vi "Autonomous Mode.vi"(0 "Drive Motors":string="RobotDrive", 1 "Ball Holders":string="RobotDrive", 5 "B.Pick up":string="My Motor RefNum", 7 "A.Pick up":string="My Solenoid RefNum", 9 "Shooter":string="My Motor RefNum", 11 "Inverted Shooter":string="My Motor RefNum") -> ()   [LabVIEW 2013]
uses:
  <vilib>/Rock Robotics/WPI/Solenoid/WPI_SolenoidValue.ctl
  <vilib>/Rock Robotics/WPI/RobotDrive/WPI_RobotDriveGetSetRefNum.vi
  <vilib>/Rock Robotics/WPI/Solenoid/Deprecated/WPI_SolenoidGetBool.vi
  <vilib>/Rock Robotics/WPI/Solenoid/WPI_SolenoidSetEnum.vi
  Ultrasonic Sensor.vi
  <vilib>/Rock Robotics/WPI/RobotDrive/WPI_RobotDriveArcadeDrive_Standard(NoSaturation).vi
panel:
  in  "Auton Shot 2":string="AUTON-Shot"
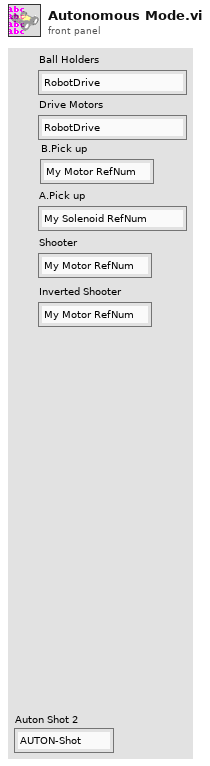
[diagram p1: front panel]
types:
  T1 = typedef "WPI_MotorControlDeviceRef.ctl" = cluster{"DeviceStatus":errorcluster, "Type":enum16{"PWM", "CAN"}, "PWM":cluster{"Digital Module":T2, "PWM Channel":T3, "DeadBand":T4}, "CAN":cluster{"Device Number":u8, "Control Mode":T5, "Semaphore":T6, "Max Vout":dbl}, "Invert":bool, "TransformRef":T7, "InvTransformRef":T7}
  T2 = typedef "FPGA_TypedefDigitalModule.ctl" = enum16{"Digital Module 1", "Digital Module 2"}
  T3 = typedef "FPGA_DIOPWMChannel.ctl" = enum8{"PWM 1", "PWM 2", "PWM 3", "PWM 4", "PWM 5", "PWM 6", "PWM 7", "PWM 8", "PWM 9", "PWM 10", "Invalid"}
  T4 = typedef "WPI_PWMDeadband.ctl" = cluster{"Name":string, "maxPositivePwm":i32, "minPositivePwm":i32, "centerPwm":i32, "maxNegativePwm":i32, "minNegativePwm":i32, "angularRange":u16}
  T5 = typedef "WPI_CANJaguar_ControlMode.ctl" = enum8{"Percent VBus", "Current", "Speed", "Position", "Voltage"}
  T6 = typedef "Semaphore RefNum" = refnum<k1>
  T7 = typedef "WPI_PWMTransform_ConPane.ctl" = refnum<vi>
  T8 = typedef "WPI_SolenoidDevRef.ctl" = cluster{"DevStatus":errorcluster, "Solenoid Module":T9, "Forward Solenoid Channel":T10, "Reverse Solenoid Channel":T10}
  T9 = typedef "FPGA_TypedefSolenoidModule.ctl" = enum16{"Solenoid Module 1", "Solenoid Module 2"}
  T10 = typedef "WPI_SolenoidChannel.ctl" = enum8{"Solenoid 1", "Solenoid 2", "Solenoid 3", "Solenoid 4", "Solenoid 5", "Solenoid 6", "Solenoid 7", "Solenoid 8", "Invalid"}
  T11 = typedef "WPI_RobotDriveDevRef.ctl" = cluster{"DevStatus":errorcluster, "Motors[]":T1[], "Square Inputs":bool, "Max Output":dbl, "Isochronous":bool}
  T12 = typedef "WPI_SolenoidValue.ctl" = enum16{"Off", "On", "Forward", "Reverse"}
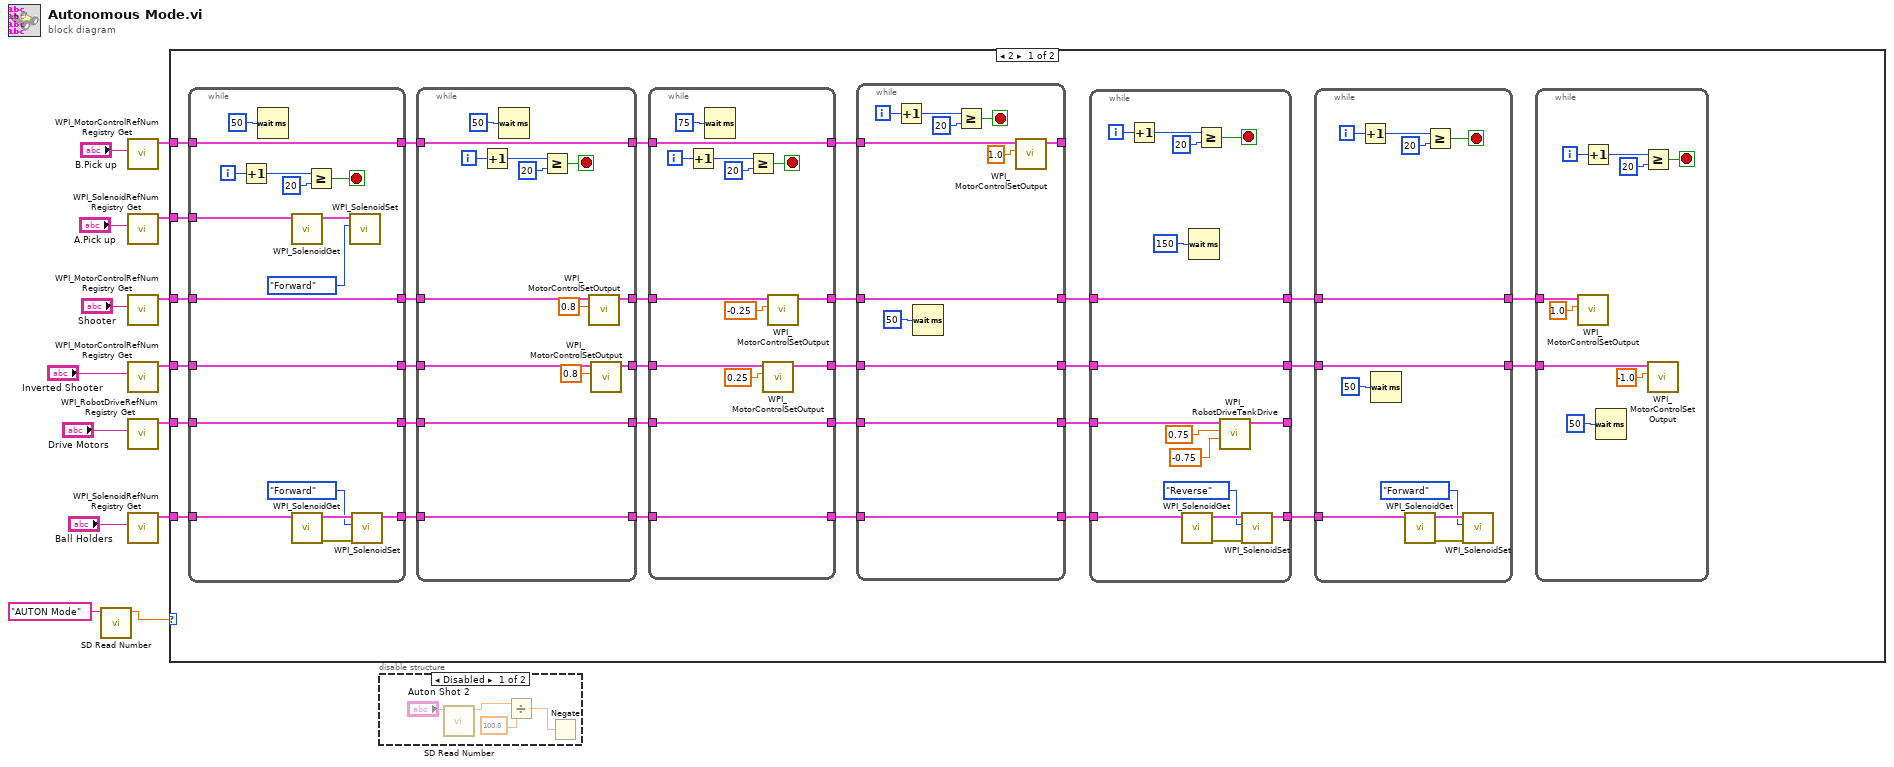
[diagram p0: block diagram]
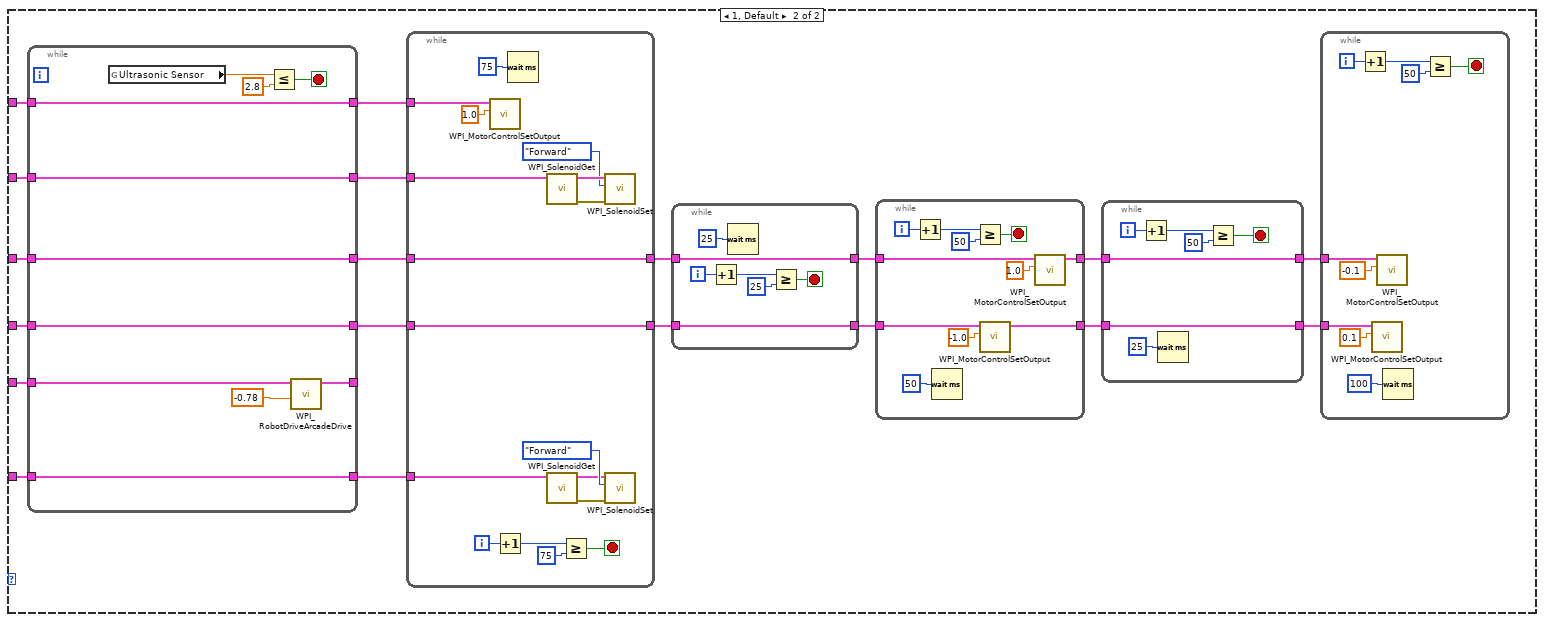
[diagram p3: hidden frame]
diagram:
  n1 = call <vilib>:"SD Read Number.vi"("Name"="AUTON Mode") -> ("Numeric"=w2:dbl)  [unwired: 8 in, 2 out]
  n2 = call <vilib>:"WPI_MotorControlRefNum Registry Get.vi"("refnum name"="B.Pick up") -> ("MotorControlDevRef"=w5:T1)  [unwired: 9 in, 1 out]
  n3 = call <vilib>:"WPI_SolenoidRefNum Registry Get.vi"("refnum name"="A.Pick up") -> ("SolenoidDevRef"=w11:T8)  [unwired: 9 in, 1 out]
  n4 = call <vilib>:"WPI_MotorControlRefNum Registry Get.vi"("refnum name"="Shooter") -> ("MotorControlDevRef"=w7:T1)  [unwired: 9 in, 1 out]
  n5 = call <vilib>:"WPI_MotorControlRefNum Registry Get.vi"("refnum name"="Inverted Shooter") -> ("MotorControlDevRef"=w6:T1)  [unwired: 9 in, 1 out]
  n6 = call <vilib>:"WPI_RobotDriveRefNum Registry Get.vi"("refnum name"="Drive Motors") -> ("RobotDriveDevRef"=w14:T11)  [unwired: 9 in, 1 out]
  n7 = call <vilib>:"WPI_SolenoidRefNum Registry Get.vi"("refnum name"="Ball Holders") -> ("SolenoidDevRef"=w3:T8)  [unwired: 9 in, 1 out]
  n8 = case shown="2" w2 {
    tunnel: w14 -> [w42 w156]
    tunnel: w11 -> [w44 w155]
    tunnel: w7 -> [w41 w154]
    tunnel: w6 -> [w40 w153]
    tunnel: w5 -> [w39 w152]
    tunnel: w3 -> [w43 w139]
    frame 2 {
      n9 = while {
        tunnel: w44 -> [w137]
        tunnel: w43 -> [w128]
        tunnel: [w134] -> w35
        tunnel: w42 -> [w134]
        tunnel: [w133] -> w38
        tunnel: w41 -> [w133]
        tunnel: [w132] -> w37
        tunnel: w40 -> [w132]
        tunnel: [w131] -> w36
        tunnel: w39 -> [w131]
        tunnel: [w126] -> w23
        i -> [w125]
        stop <- w124 stop-if-true
        n10 = Increment(x=w125) -> (x+1=w123:i32)
        n11 = Wait (ms)(milliseconds to wait=u32 50) -> ()  [unwired: 1 out]
        n12 = call-poly <vilib>:"WPI_SolenoidGet.vi"("SolenoidDevRef"=w137) -> ("SolenoidDevRef"=w136:T8)  [unwired: 8 in, 2 out]
        n13 = call-poly <vilib>:"WPI_SolenoidGet.vi"("SolenoidDevRef"=w128) -> ("error out"=w130:errorcluster, "SolenoidDevRef"=w129:T8)  [unwired: 8 in, 1 out]
        n14 = Greater Or Equal?(x=w123, y=20) -> (x >= y?=w124:bool)
        n15 = call-poly <vilib>:"WPI_SolenoidSet.vi"("Value"=WPI_SolenoidValue."Forward", "SolenoidDevRef"=w136) -> ()  [unwired: 8 in, 2 out]
        n16 = call-poly <vilib>:"WPI_SolenoidSet.vi"("error in (no error)"=w130, "Value"=WPI_SolenoidValue."Forward", "SolenoidDevRef"=w129) -> ("SolenoidDevRef"=w126:T8)  [unwired: 7 in, 1 out]
      }
      n17 = while {
        tunnel: w38 -> [w120]
        tunnel: w37 -> [w119]
        tunnel: [w118] -> w32
        tunnel: [w117] -> w33
        tunnel: [w116] -> w31
        tunnel: w36 -> [w116]
        tunnel: [w115] -> w34
        tunnel: w35 -> [w115]
        tunnel: [w114] -> w22
        tunnel: w23 -> [w114]
        i -> [w113]
        stop <- w110 stop-if-true
        n18 = Increment(x=w113) -> (x+1=w112:i32)
        n19 = Wait (ms)(milliseconds to wait=u32 50) -> ()  [unwired: 1 out]
        n20 = Greater Or Equal?(x=w112, y=20) -> (x >= y?=w110:bool)
        n21 = call <vilib>:"WPI_MotorControlSetOutput.vi"("Output"=0.8, "MotorControlDevRef"=w120) -> ("MotorControlDevRef"=w117:T1)  [unwired: 7 in, 2 out]
        n22 = call <vilib>:"WPI_MotorControlSetOutput.vi"("Output"=0.8, "MotorControlDevRef"=w119) -> ("MotorControlDevRef"=w118:T1)  [unwired: 7 in, 2 out]
      }
      n23 = while {
        tunnel: w34 -> [w101]
        tunnel: w33 -> [w103]
        tunnel: w32 -> [w104]
        tunnel: w31 -> [w102]
        tunnel: [w102] -> w28
        tunnel: [w101] -> w27
        tunnel: [w100] -> w29
        tunnel: [w99] -> w30
        tunnel: w22 -> [w98]
        tunnel: [w98] -> w21
        i -> [w97]
        stop <- w94 stop-if-true
        n24 = Increment(x=w97) -> (x+1=w96:i32)
        n25 = Wait (ms)(milliseconds to wait=u32 75) -> ()  [unwired: 1 out]
        n26 = Greater Or Equal?(x=w96, y=20) -> (x >= y?=w94:bool)
        n27 = call <vilib>:"WPI_MotorControlSetOutput.vi"("Output"=0.25, "MotorControlDevRef"=w104) -> ("MotorControlDevRef"=w100:T1)  [unwired: 7 in, 2 out]
        n28 = call <vilib>:"WPI_MotorControlSetOutput.vi"("Output"=-0.25, "MotorControlDevRef"=w103) -> ("MotorControlDevRef"=w99:T1)  [unwired: 7 in, 2 out]
      }
      n29 = while {
        tunnel: w30 -> [w89]
        tunnel: w29 -> [w90]
        tunnel: w28 -> [w92]
        tunnel: w27 -> [w88]
        tunnel: [w90] -> w26
        tunnel: [w89] -> w25
        tunnel: [w88] -> w24
        tunnel: [w87] -> _
        tunnel: w21 -> [w86]
        tunnel: [w86] -> w20
        i -> [w85]
        stop <- w82 stop-if-true
        n30 = Increment(x=w85) -> (x+1=w84:i32)
        n31 = Wait (ms)(milliseconds to wait=u32 50) -> ()  [unwired: 1 out]
        n32 = Greater Or Equal?(x=w84, y=20) -> (x >= y?=w82:bool)
        n33 = call <vilib>:"WPI_MotorControlSetOutput.vi"("Output"=1.0, "MotorControlDevRef"=w92) -> ("MotorControlDevRef"=w87:T1)  [unwired: 7 in, 2 out]
      }
      n34 = while {
        tunnel: [w80] -> w17
        tunnel: w26 -> [w80]
        tunnel: w25 -> [w79]
        tunnel: [w79] -> w18
        tunnel: w24 -> [w78]
        tunnel: [w76] -> _
        tunnel: w20 -> [w75]
        tunnel: [w71] -> w19
        i -> [w70]
        stop <- w66 stop-if-true
        n35 = Increment(x=w70) -> (x+1=w69:i32)
        n36 = call-poly <vilib>:"WPI_SolenoidGet.vi"("SolenoidDevRef"=w75) -> ("error out"=w74:errorcluster, "SolenoidDevRef"=w73:T8)  [unwired: 8 in, 1 out]
        n37 = Wait (ms)(milliseconds to wait=u32 150) -> ()  [unwired: 1 out]
        n38 = Greater Or Equal?(x=w69, y=20) -> (x >= y?=w66:bool)
        n39 = call <vilib>:"WPI_RobotDriveTankDrive.vi"("Right axis value"=-0.75, "Left axis value"=0.75 ("X axis value"), "RobotDriveDevRef"=w78) -> ("RobotDriveDevRef"=w76:T11)  [unwired: 6 in, 2 out]
        n40 = call-poly <vilib>:"WPI_SolenoidSet.vi"("error in (no error)"=w74, "Value"=WPI_SolenoidValue."Reverse", "SolenoidDevRef"=w73) -> ("SolenoidDevRef"=w71:T8)  [unwired: 7 in, 1 out]
      }
      n41 = while {
        tunnel: w19 -> [w64]
        tunnel: w18 -> [w60]
        tunnel: w17 -> [w59]
        tunnel: [w60] -> w16
        tunnel: [w59] -> w15
        i -> [w57]
        stop <- w54 stop-if-true
        n42 = Increment(x=w57) -> (x+1=w58:i32)
        n43 = Wait (ms)(milliseconds to wait=u32 50) -> ()  [unwired: 1 out]
        n44 = call-poly <vilib>:"WPI_SolenoidGet.vi"("SolenoidDevRef"=w64) -> ("error out"=w63:errorcluster, "SolenoidDevRef"=w62:T8)  [unwired: 8 in, 1 out]
        n45 = Greater Or Equal?(x=w58, y=20) -> (x >= y?=w54:bool)
        n46 = call-poly <vilib>:"WPI_SolenoidSet.vi"("error in (no error)"=w63, "Value"=WPI_SolenoidValue."Forward", "SolenoidDevRef"=w62) -> ()  [unwired: 7 in, 2 out]
      }
      n47 = while {
        tunnel: w16 -> [w53]
        tunnel: w15 -> [w52]
        i -> [w49]
        stop <- w46 stop-if-true
        n48 = call <vilib>:"WPI_MotorControlSetOutput.vi"("Output"=1.0, "MotorControlDevRef"=w53) -> ()  [unwired: 7 in, 3 out]
        n49 = Increment(x=w49) -> (x+1=w48:i32)
        n50 = Wait (ms)(milliseconds to wait=u32 50) -> ()  [unwired: 1 out]
        n51 = Greater Or Equal?(x=w48, y=20) -> (x >= y?=w46:bool)
        n52 = call <vilib>:"WPI_MotorControlSetOutput.vi"("Output"=-1.0, "MotorControlDevRef"=w52) -> ()  [unwired: 7 in, 3 out]
      }
    }
    frame 1, Default {
      n53 = while {
        tunnel: [w218] -> _
        tunnel: w156 -> [w217]
        tunnel: w155 -> [w216]
        tunnel: [w216] -> w151
        tunnel: [w215] -> w148
        tunnel: w154 -> [w215]
        tunnel: [w214] -> w149
        tunnel: w153 -> [w214]
        tunnel: [w213] -> w150
        tunnel: w152 -> [w213]
        tunnel: w139 -> [w208]
        tunnel: [w208] -> w138
        stop <- w210 stop-if-true
        n54 = global read "Ultrasonic Sensor.vi" "Ultrasonic Sensor"() -> (w212:dbl)
        n55 = Less Or Equal?(x=w212, y=2.8) -> (x <= y?=w210:bool)
        n56 = call-poly <vilib>:"WPI_RobotDriveArcadeDrive.vi"("Y axis value"=-0.78, "RobotDriveDevRef"=w217) -> ("RobotDriveDevRef"=w218:T11)  [unwired: 7 in, 2 out]
      }
      n57 = while {
        tunnel: w151 -> [w207]
        tunnel: w150 -> [w199]
        tunnel: w149 -> [w195]
        tunnel: w148 -> [w196]
        tunnel: [w196] -> w147
        tunnel: [w195] -> w146
        tunnel: w138 -> [w191]
        i -> [w206]
        stop <- w203 stop-if-true
        n58 = call <vilib>:"WPI_MotorControlSetOutput.vi"("Output"=1.0, "MotorControlDevRef"=w199) -> ()  [unwired: 7 in, 3 out]
        n59 = Increment(x=w206) -> (x+1=w205:i32)
        n60 = Wait (ms)(milliseconds to wait=u32 75) -> ()  [unwired: 1 out]
        n61 = call-poly <vilib>:"WPI_SolenoidGet.vi"("SolenoidDevRef"=w207) -> ("error out"=w202:errorcluster, "SolenoidDevRef"=w201:T8)  [unwired: 8 in, 1 out]
        n62 = call-poly <vilib>:"WPI_SolenoidGet.vi"("SolenoidDevRef"=w191) -> ("error out"=w192:errorcluster, "SolenoidDevRef"=w193:T8)  [unwired: 8 in, 1 out]
        n63 = Greater Or Equal?(x=w205, y=75) -> (x >= y?=w203:bool)
        n64 = call-poly <vilib>:"WPI_SolenoidSet.vi"("error in (no error)"=w202, "Value"=WPI_SolenoidValue."Forward", "SolenoidDevRef"=w201) -> ()  [unwired: 7 in, 2 out]
        n65 = call-poly <vilib>:"WPI_SolenoidSet.vi"("error in (no error)"=w192, "Value"=WPI_SolenoidValue."Forward", "SolenoidDevRef"=w193) -> ()  [unwired: 7 in, 2 out]
      }
      n66 = while {
        tunnel: [w186] -> w145
        tunnel: w147 -> [w186]
        tunnel: w146 -> [w185]
        tunnel: [w185] -> w144
        i -> [w187]
        stop <- w188 stop-if-true
        n67 = Increment(x=w187) -> (x+1=w189:i32)
        n68 = Wait (ms)(milliseconds to wait=u32 25) -> ()  [unwired: 1 out]
        n69 = Greater Or Equal?(x=w189, y=25) -> (x >= y?=w188:bool)
      }
      n70 = while {
        tunnel: w145 -> [w178]
        tunnel: w144 -> [w179]
        tunnel: [w175] -> w143
        tunnel: [w174] -> w142
        i -> [w183]
        stop <- w180 stop-if-true
        n71 = Increment(x=w183) -> (x+1=w182:i32)
        n72 = Wait (ms)(milliseconds to wait=u32 50) -> ()  [unwired: 1 out]
        n73 = Greater Or Equal?(x=w182, y=50) -> (x >= y?=w180:bool)
        n74 = call <vilib>:"WPI_MotorControlSetOutput.vi"("Output"=-1.0, "MotorControlDevRef"=w179) -> ("MotorControlDevRef"=w174:T1)  [unwired: 7 in, 2 out]
        n75 = call <vilib>:"WPI_MotorControlSetOutput.vi"("Output"=1.0, "MotorControlDevRef"=w178) -> ("MotorControlDevRef"=w175:T1)  [unwired: 7 in, 2 out]
      }
      n76 = while {
        tunnel: w143 -> [w166]
        tunnel: w142 -> [w167]
        tunnel: [w167] -> w141
        tunnel: [w166] -> w140
        i -> [w170]
        stop <- w169 stop-if-true
        n77 = Increment(x=w170) -> (x+1=w172:i32)
        n78 = Wait (ms)(milliseconds to wait=u32 25) -> ()  [unwired: 1 out]
        n79 = Greater Or Equal?(x=w172, y=50) -> (x >= y?=w169:bool)
      }
      n80 = while {
        tunnel: w141 -> [w165]
        tunnel: w140 -> [w164]
        i -> [w161]
        stop <- w160 stop-if-true
        n81 = Increment(x=w161) -> (x+1=w162:i32)
        n82 = call <vilib>:"WPI_MotorControlSetOutput.vi"("Output"=0.1, "MotorControlDevRef"=w165) -> ()  [unwired: 7 in, 3 out]
        n83 = call <vilib>:"WPI_MotorControlSetOutput.vi"("Output"=-0.1, "MotorControlDevRef"=w164) -> ()  [unwired: 7 in, 3 out]
        n84 = Wait (ms)(milliseconds to wait=u32 100) -> ()  [unwired: 1 out]
        n85 = Greater Or Equal?(x=w162, y=50) -> (x >= y?=w160:bool)
      }
    }
  }
  n86 = disable-structure shown="Disabled" {
    frame Disabled {
      n87 = call <vilib>:"SD Read Number.vi"("Name"="Auton Shot 2") -> ("Numeric"=w220:dbl)  [unwired: 8 in, 2 out]
      n88 = Divide(x=w220, y=100.0) -> (x/y=w222:dbl)
      n89 = Negate(x=w222) -> ()  [unwired: 1 out]
    }
    frame Enabled {
    }
  }
